vi "signal_gen_test.vi"() -> ()   [LabVIEW 2025]
panel:
  out "Waveform Graph":dbl[](graph)
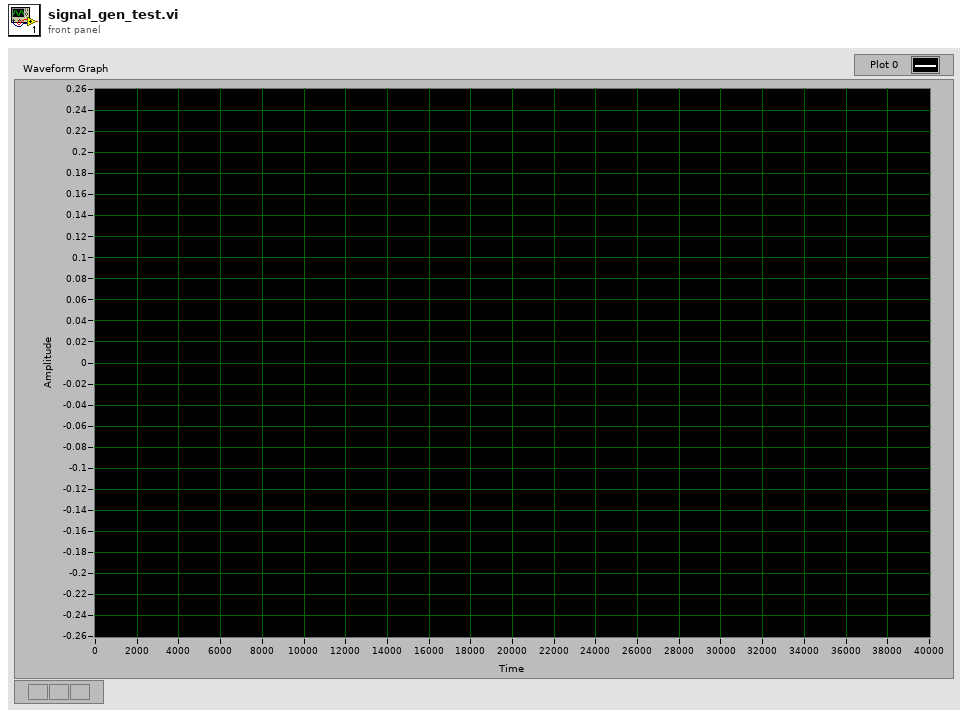
[diagram p1: front panel]
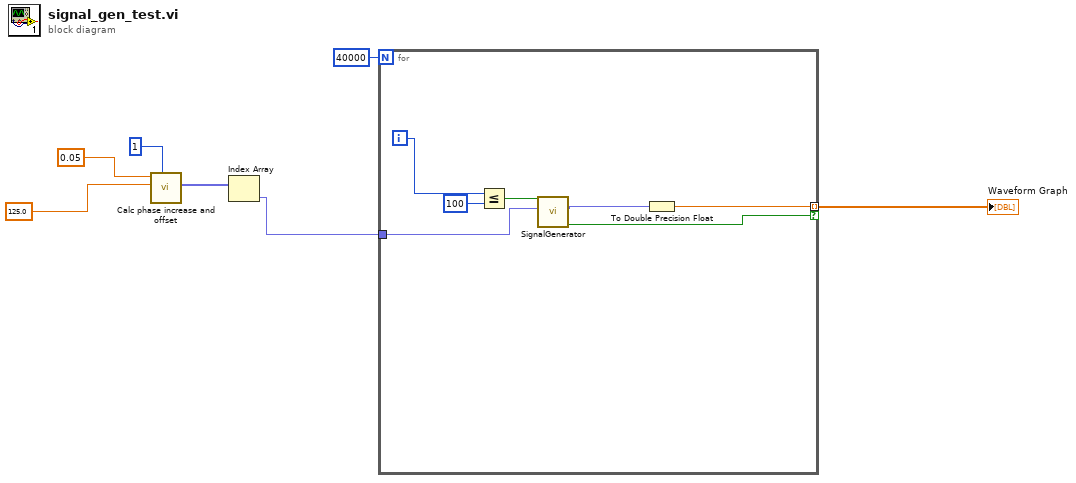
[diagram p0: block diagram]
diagram:
  n1 = call "Calc phase increase and offset.vi"("# of DDS"=1, "fclk (MHz)"=125.0, "f_generated (MHz)"=0.05) -> ("Phase out"=w2:fxp<+,64,64>[])  [unwired: 6 in, 2 out]
  n2 = Index Array(array=w2) -> (element=w1:fxp<+,64,64>)  [unwired: 1 in]
  n3 = for {
    N: 40000 -> [_]
    tunnel: [w13] -> w6 mode=indexing if=w9
    tunnel: w1 -> [w8]
    i -> [w12]
    n4 = Less Or Equal?(x=w12, y=100) -> (x <= y?=w10:bool)
    n5 = call "SignalGenerator.vi"("phase"=w8, "Reset"=w10) -> ("data_valid"=w9:bool, "Sin"=w14:fxp<+/-,18,1>)  [unwired: 7 in, 1 out]
    n6 = To Double Precision Float(number=w14) -> (double precision float=w13:dbl)
  }
  "Waveform Graph" <- w6
